vi "WAM_SN_Prompt.vi"(0 "Enable":bool=TRUE, 11 "error in (no error)":errorcluster, 12 "Rev_suffix":string) -> (1 "Bar Code":string, 2 "BarCodeInfo":string, 3 "BC_MSN":string, 4 "cancelled?(t)":bool, 6 "LotID":string, 10 "rev_c?(t)":bool, 13 "BC_ESN":string, 14 "Revision":string, 15 "error out":errorcluster)   [LabVIEW 2018]
uses:
  Initialize References/Sequence Globals.vi
panel:
  out "Leidos_SN?(t)":bool
  out "Company":string
  out "Rage PN":string
  out "match substring":string
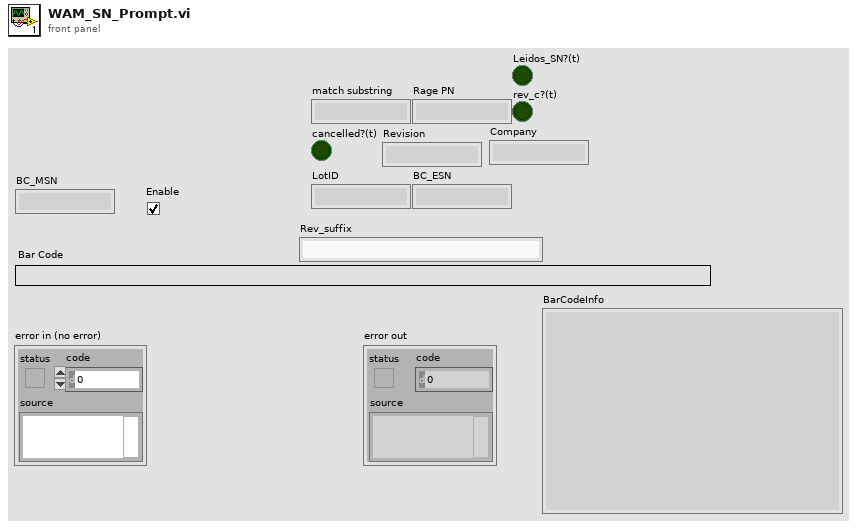
[diagram p1: front panel]
types:
  T1 = enum16{"open", "replace", "create", "open or create", "replace or create", "replace or create with confirmation"}
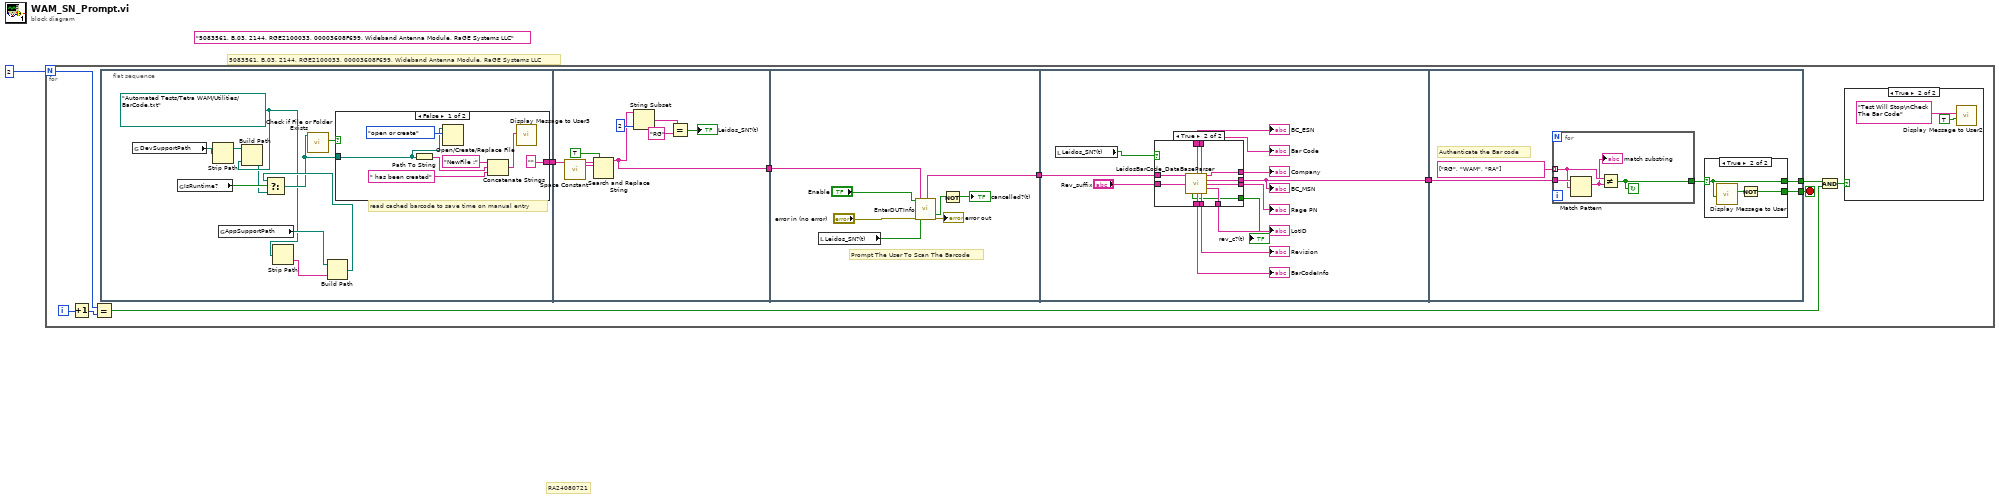
[diagram p0: block diagram]
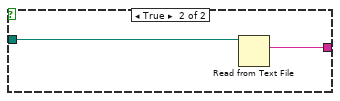
[diagram p3: hidden frame]
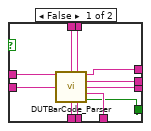
[diagram p4: hidden frame]
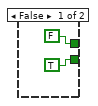
[diagram p5: hidden frame]
diagram:
  (unwired) "5083561, B.03, 2144, RGE2100033, 00003608F699, Wideband Antenna Module, RaGE Systems LLC" ("Bar Code")
  # "RA24080721"
  # "5083561, B.03, 2144, RGE2100033, 00003608F699, Wideband Antenna Module, RaGE Systems LLC"
  n1 = for {
    N: 2 -> [w9]
    i -> [w10]
    stop <- w7 stop-if-true
    n2 = Increment(x=w10) -> (x+1=w8:i32)
    n3 = Equal?(x=w9, y=w8) -> (x = y?=w5:bool)
    n4 = flat-sequence {
      tunnel: [w25] -> w3
      tunnel: w3 -> [w42]
      tunnel: [w38] -> w2
      tunnel: [w49] -> w12
      tunnel: w2 -> [w44]
      tunnel: w12 -> [w62]
      tunnel: [w54] -> w11
      tunnel: w11 -> [w89]
      tunnel: [w87] -> w7
      tunnel: [w85] -> w4
      frame #0 {
        w16 = path "Automated Tests/Tetra WAM/Utilities/BarCode.txt" ("file (use dialog)")
        # "read cached barcode to save time on manual entry"
        n5 = global read "Sequence Globals.vi" "DevSupportPath"() -> (w18:path)
        n6 = global read "Sequence Globals.vi" "IsRuntime?"() -> (w20:bool)
        n7 = Strip Path(path=w18) -> (stripped path=w17:path)  [unwired: 1 out]
        n8 = global read "Sequence Globals.vi" "AppSupportPath"() -> (w22:path)
        n9 = Build Path(base path=w17, name or relative path=w16) -> (appended path=w15:path)
        n10 = Strip Path(path=w16) -> (name=w23:string)  [unwired: 1 out]
        n11 = Build Path(base path=w22, name or relative path=w23) -> (appended path=w21:path)
        n12 = Select(t=w21, s=w20, f=w15) -> (s? t:f=w19:path)
        n13 = call <vilib>:"Check if File or Folder Exists.vi"("path"=w19) -> ("file or folder exists?"=w24:bool)  [unwired: 8 in, 2 out]
        n14 = case shown="False" w24 {
          tunnel: w19 -> [w28 w34]
          tunnel: ["" w33] -> w25
          frame False {
            n15 = Path To String(path=w28) -> (string=w27:string)
            n16 = Open/Create/Replace File(file path (use dialog)=w28, operation (0:open)=T1."open or create") -> ()  [unwired: 4 in, 3 out]
            n17 = Concatenate Strings("NewFile :" ("Message"), w27, " has been created" ("string")) -> (w29:string)
            n18 = call "Display Message to User3"("Message"=w29) -> ()  [unwired: 9 in, 2 out]
          }
          frame True {
            n19 = Read from Text File(file (use dialog)=w34) -> (text=w33:string)  [unwired: 3 in, 3 out]
          }
        }
      }
      frame #1 {
        n20 = call <vilib>:"Space Constant.vi"() -> ("String"=w41:string)
        n21 = Search and Replace String(replace all?=TRUE ("replace all? (F)"), input string=w42, search string=w41) -> (result string=w38:string)  [unwired: 5 in, 3 out]
        n22 = String Subset(string=w38, length (rest)=2 ("length (rest)")) -> (substring=w37:string)  [unwired: 1 in]
        n23 = Equal?(x=w37, y="RG") -> (x = y?=→"Leidos_SN?(t)":bool)
      }
      frame #2 {
        # "Prompt The User To Scan The Barcode"
        n24 = local read "Leidos_SN?(t)"() -> (w43:bool)
        n25 = call "EnterDUTInfo.vi"("Enable"="Enable", "error in (no error)"="error in (no error)", "InputData"=w44, "Leidos_sn(t)"=w43) -> ("DUT INFO"=w49:string, "OK"=w46:bool, "error out"=→"error out":errorcluster)  [unwired: 7 in, 6 out]
        n26 = Not(x=w46) -> (.not. x?=→"cancelled?(t)":bool)
      }
      frame #3 {
        n27 = local read "Leidos_SN?(t)"() -> (w52:bool)
        n28 = case shown="True" w52 {
          tunnel: w62 -> [w73 w84]
          tunnel: [w72 w83] -> w61
          tunnel: [w71 w82] -> w60
          tunnel: [w70 w81] -> w59
          tunnel: [w69 w80] -> w58
          tunnel: [w68 w79] -> w57
          tunnel: [w67 w78] -> w56
          tunnel: [w66 w77] -> w55
          tunnel: [w65 w76] -> w54
          tunnel: "Rev_suffix" -> [w64 w75]
          tunnel: [w63 w74] -> w51
          frame False {
            n29 = call "DUTBarCode_Parser.vi"("DUT INFO"=w73, "Rev_suffix"=w64) -> ("BC_ESN"=w66:string, "Bar Code"=w72:string, "Company"=w71:string, "BC_MSN"=w65:string, "Rage PN"=w70:string, "LotID"=w67:string, "BarCodeInfo"=w68:string, "Revision"=w69:string, "rev_c?(t)"=w63:bool)  [unwired: 4 in, 1 out]
          }
          frame True {
            n30 = call "LeidosBarCode_DataBaseParser.vi"("BarCode_In"=w84, "Rev_suffix"=w75) -> ("BC_ESN"=w77:string, "BarCode_Out"=w83:string, "Company"=w82:string, "BC_MSN"=w76:string, "Rage PN"=w81:string, "LotID"=w78:string, "rev_c?(t)"=w74:bool, "BarCodeInfo"=w79:string, "Revision"=w80:string)  [unwired: 3 in, 2 out]
          }
        }
        "BC_MSN" <- w54
        "Rage PN" <- w59
        "Revision" <- w58
        "LotID" <- w56
        "BC_ESN" <- w55
        "Company" <- w60
        "BarCodeInfo" <- w57
        "Bar Code" <- w61
        "rev_c?(t)" <- w51
      }
      frame #4 {
        # "Authenticate the Bar code"
        n31 = for {
          tunnel: w89 -> [w93]
          tunnel: string[] ["RG", "WAM", "RA"] ("regular expression") -> [w92] mode=indexing
          tunnel: [w90] -> w86
          stop <- w90 continue-if-true
          n32 = Match Pattern(string=w93, regular expression=w92) -> (match substring=w91:string)  [unwired: 1 in, 3 out]
          "match substring" <- w91
          n33 = Not Equal?(x=w92, y=w91) -> (x != y?=w90:bool)
        }
        n34 = case shown="True" w86 {
          selector: w86 -> [_ w96]
          tunnel: [TRUE w97] -> w87
          tunnel: [FALSE w96] -> w85
          frame False {
          }
          frame True {
            n35 = call "Display Message to User"("Enable"=w96) -> ("OK"=w98:bool)  [unwired: 9 in, 1 out]
            n36 = Not(x=w98) -> (.not. x?=w97:bool)
          }
        }
      }
    }
    n37 = And(x=w4, y=w5) -> (x .and. y?=w6:bool)
    n38 = case shown="True" w6 {
      frame False {
      }
      frame True {
        n39 = call "Display Message to User2"("Enable"=TRUE, "Message"="Test Will Stop\nCheck The Bar Code") -> ()  [unwired: 8 in, 2 out]
      }
    }
  }
